vi "PH_ImageCoG_Plotter.evt call Read Cali Data.vi"(0 "i ref in":refnum<vi>, 5 "error in":errorcluster) -> (14 "i ref out":refnum<vi>, 19 "error out":errorcluster)   [LabVIEW 2014, in "PH_ImageCoG_Plotter.lvlib"]
doc: "This VI calls the event case \"ReadCaliData\" by a simple call."
uses:
  PH_ImageCoG_Plotter.lvlib
  CSCore/CSSystem/CSSystemLib/CSSystemLib.lvlib
  CSCore/BaseProcess/BaseProcess.lvlib
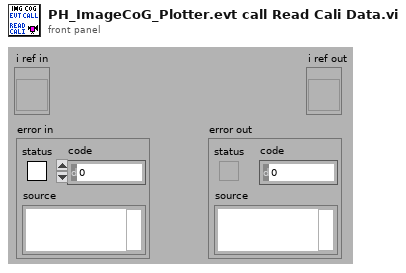
[diagram p1: front panel]
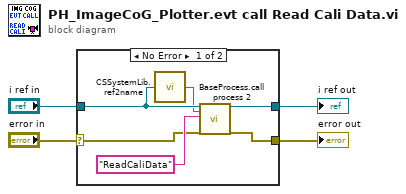
[diagram p0: block diagram]
diagram:
  n1 = case shown="No Error" "error in" {
    selector: "error in" -> [w5 w11]
    tunnel: [w9 w12] -> w4
    tunnel: [w8 w11] -> w3
    tunnel: "i ref in" -> [w7 w12]
    frame No Error {
      n2 = call "CSSystemLib.ref2name.vi"("obj refnum"=w7) -> ("name"=w6:string)
      n3 = call "BaseProcess.call process 2.vi"("i ref in"=w7, "Object"=w6, "Selector"="ReadCaliData", "error in (no error)"=w5) -> ("i ref out"=w9:refnum<vi>, "error out"=w8:errorcluster)  [unwired: 14 in]
    }
    frame Error {
    }
  }
  "i ref out" <- w4
  "error out" <- w3
